vi "GPS~Logger.vi"(2 "file path (use dialog)":path, 3 "baud rate (115200)":u32=115200, 4 "stop":bool, 5 "VISA resource name":refnum<visa-resource-name>) -> (0 "Longitude":dbl format="%#_15g", 1 "Lattitude":dbl format="%#_15g")   [LabVIEW 2010]
uses:
  <vilib>/robotics/Controls/Attitude Indicator/Attitude Indicator.xctl
  <vilib>/robotics/Controls/Compass Indicator/Compass Indicator.xctl
  <vilib>/Instr/_visa.llb/VISA Set IO Buffer Mask.ctl
  <vilib>/Instr/_visa.llb/VISA Configure Serial Port (Instr).vi
panel:
  out "Bearing":dbl
  out "Speed":dbl(knob) scale=0.0..40.0
  out "LiPo":i32(slide) scale=9.0..12.6
  out "GPS Time":string
  out "Servo Roll":string
  out "Battery Voltage":dbl
  out "Distance to Waypoint":string
  out "Waypoint Number":string
  out "Flight Mode":string
  out "Compass Indicator":dbl(xcontrol)
  out "Attitude Indicator":cluster{"Roll":dbl, "Pitch":dbl}(xcontrol)
  out "Message Text":string
  in  "Tab Control":enum32{"Connectivity", "Attitude", "GPS"}(tab)
  out "error out":errorcluster {"code" format="%f"}
  out "Roll":string
  out "Pitch":string
  out "Throttle":string
  out "Airspeed":string
  out "Roll Pitch":cluster{dbl, dbl}
  out "YawNum":dbl
  out "ALT":string
  out "ALH":string
  out "BER":string
  out "CRT":string
  out "SPD":string
  out "CRS":string
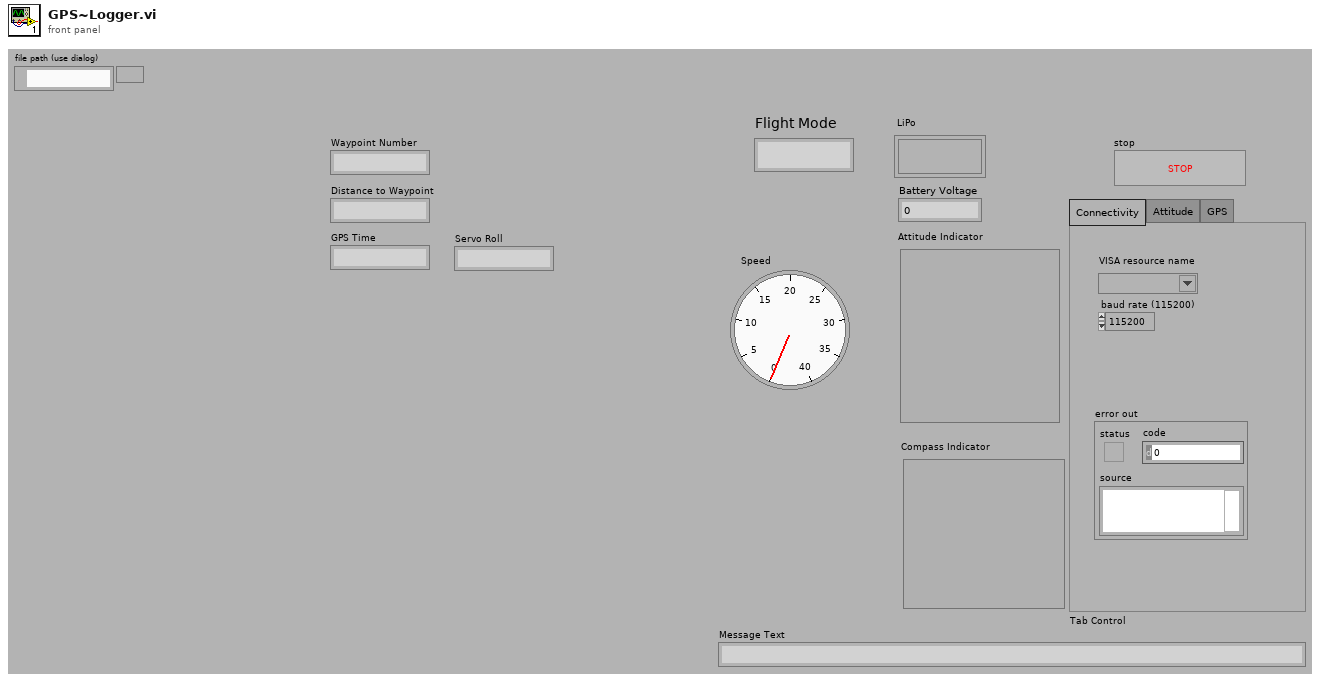
[diagram p1: front panel]
types:
  T1 = typedef "VISA Set IO Buffer Mask.ctl" = u16
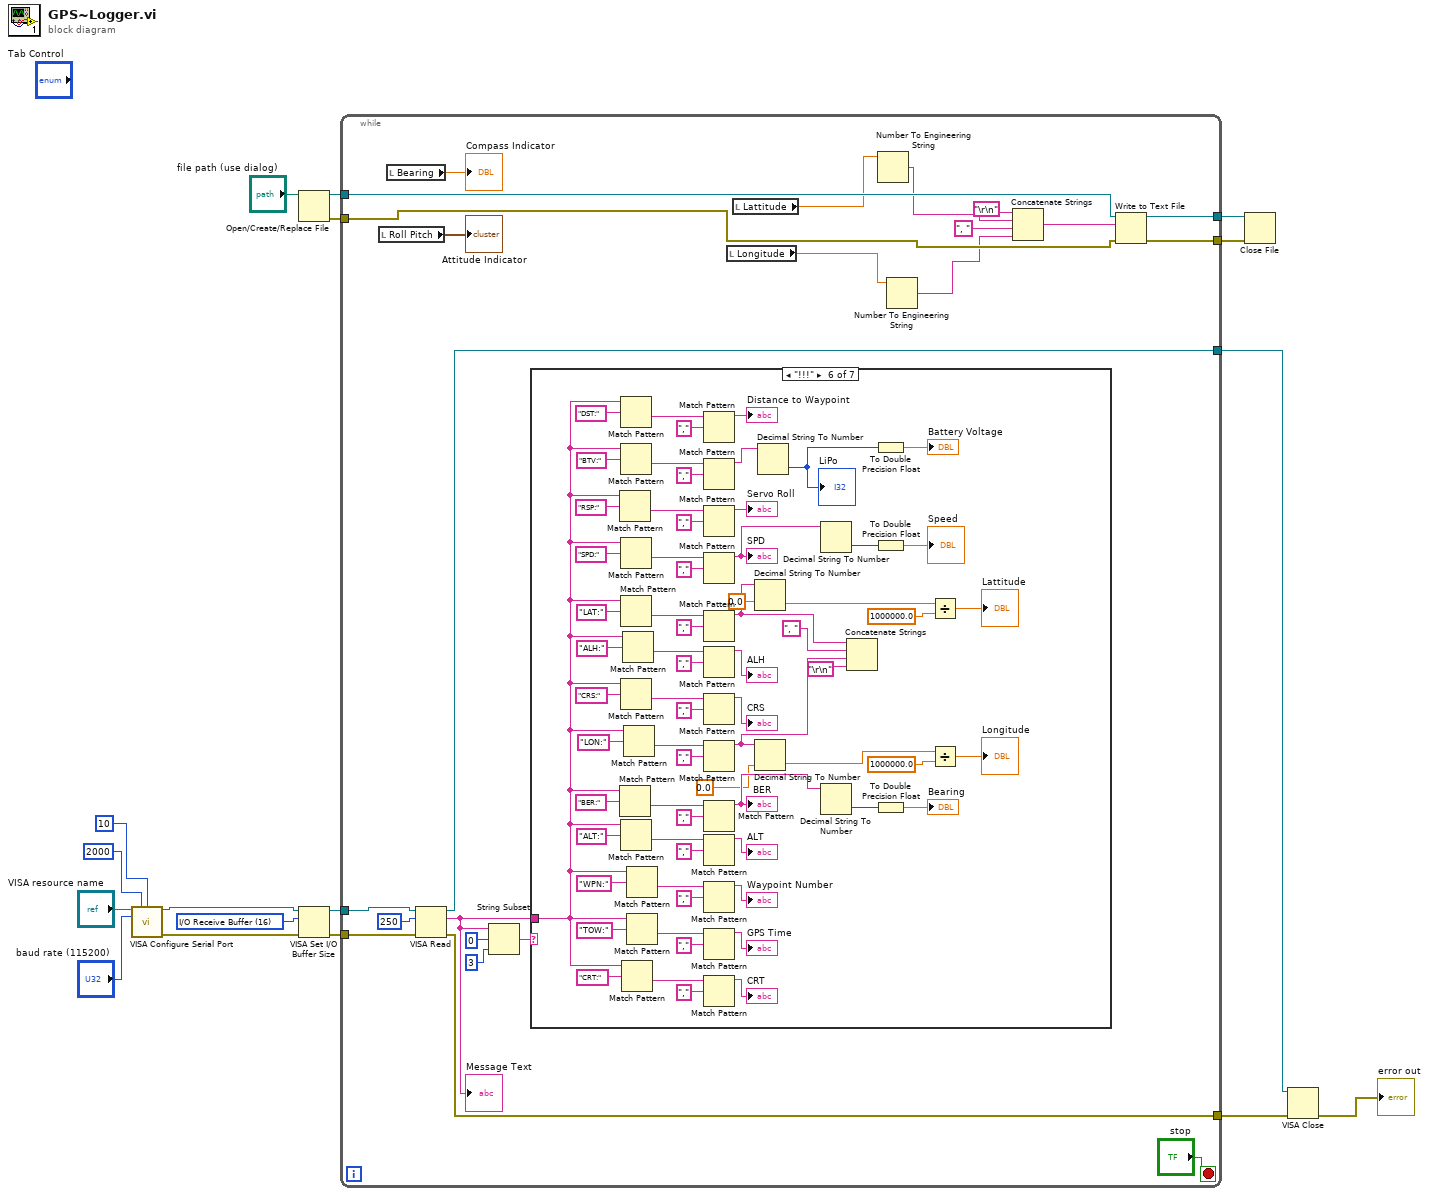
[diagram p0: block diagram]
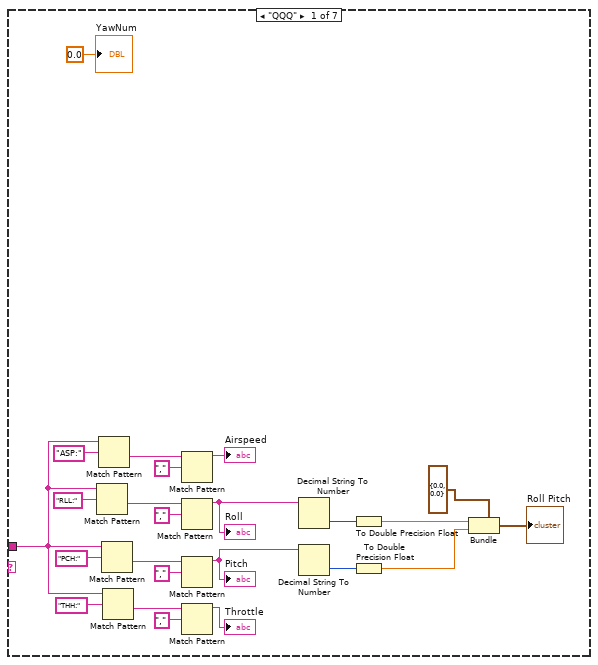
[diagram p2: hidden frame]
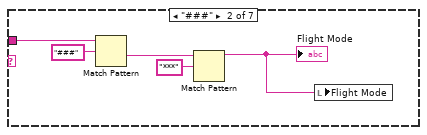
[diagram p3: hidden frame]
diagram:
  w12 = T1 16 items=["I/O Receive Buffer"=16, "I/O Transmit Buffer"=32, "I/O Receive and Transmit Buffer"=48] ("Mask")
  n1 = call-poly "VISA Configure Serial Port"("VISA resource name"="VISA resource name", "timeout (10sec)"=u32 2000, "termination char\n(0xA = '\\n' = LF)"=u8 10 ("termination char\n(0xA = '\\n' = LF)"), "baud rate (9600)"="baud rate (115200)") -> ("VISA resource name out"=w13:refnum<visa-resource-name>, "error out"=w7:errorcluster)  [unwired: 10 in]
  n2 = Open/Create/Replace File(file path (use dialog)="file path (use dialog)") -> (refnum out=w5:refnum<file>, error out=w1:errorcluster)  [unwired: 5 in, 1 out]
  n3 = VISA Set I/O Buffer Size(VISA resource name=w13, mask (16)=w12, error in (no error)=w7) -> (VISA resource name out=w11:refnum<visa-resource-name>, error out=w8:errorcluster)  [unwired: 1 in]
  n4 = while {
    tunnel: w11 -> [w40]
    tunnel: [w38] -> w10
    tunnel: [w37] -> w9
    tunnel: w8 -> [w36]
    tunnel: w5 -> [w28]
    tunnel: [w27] -> w3
    tunnel: [w24] -> w2
    tunnel: w1 -> [w23]
    stop <- "stop" stop-if-true
    n5 = local read "Roll Pitch"() -> (→"Attitude Indicator":cluster{dbl, dbl})
    n6 = local read "Bearing"() -> (→"Compass Indicator":dbl)
    n7 = VISA Read(VISA resource name=w40, byte count=u32 250, error in (no error)=w36) -> (VISA resource name out=w38:refnum<visa-resource-name>, read buffer=w30:string, error out=w37:errorcluster)  [unwired: 1 out]
    "Message Text" <- w30
    n8 = String Subset(string=w30, offset (0)=0, length (rest)=3 ("length (rest)")) -> (substring=w29:string)
    n9 = case shown="\"!!!\"" w29 {
      tunnel: w30 -> [w42 w69 _ _ _ w90 _]
      frame "QQQ" {
        n10 = Match Pattern(string=w42, regular expression="RLL:") -> (after substring=w63:string)  [unwired: 4 out]
        n11 = Match Pattern(string=w42, regular expression="ASP:") -> (after substring=w54:string)  [unwired: 4 out]
        n12 = Match Pattern(string=w42, regular expression="PCH:") -> (after substring=w60:string)  [unwired: 4 out]
        n13 = Match Pattern(string=w42, regular expression="THH:") -> (after substring=w57:string)  [unwired: 4 out]
        n14 = Match Pattern(string=w54, regular expression=",") -> (before substring=→"Airspeed":string)  [unwired: 4 out]
        n15 = Match Pattern(string=w63, regular expression=",") -> (before substring=w45:string)  [unwired: 4 out]
        "Roll" <- w45
        n16 = Match Pattern(string=w60, regular expression=",") -> (before substring=w44:string)  [unwired: 4 out]
        "Pitch" <- w44
        n17 = Match Pattern(string=w57, regular expression=",") -> (before substring=→"Throttle":string)  [unwired: 4 out]
        n18 = Decimal String To Number(string=w45) -> (number=w51:i32)  [unwired: 2 in, 1 out]
        n19 = Decimal String To Number(string=w44) -> (number=w50:i32)  [unwired: 2 in, 1 out]
        n20 = To Double Precision Float(number=w51) -> (double precision float=w48:dbl)
        n21 = To Double Precision Float(number=w50) -> (double precision float=w49:dbl)
        n22 = Bundle(cluster=cluster{dbl, dbl} {0.0, 0.0} ("Cluster"), w48, w49) -> (→"Roll Pitch":cluster{dbl, dbl})
        "YawNum" <- 0.0 ("YawNum")
      }
      frame "###" {
        n23 = Match Pattern(string=w69, regular expression="###") -> (after substring=w67:string)  [unwired: 1 in, 3 out]
        n24 = Match Pattern(string=w67, regular expression="***") -> (before substring=w65:string)  [unwired: 1 in, 3 out]
        "Flight Mode" <- w65
        n25 = local write "Flight Mode"(w65) -> ()
      }
      frame "%%%" {
      }
      frame "XXX" {
      }
      frame "PPP" {
      }
      frame "!!!" {
        n26 = Match Pattern(string=w90, regular expression="RSP:") -> (after substring=w97:string)  [unwired: 4 out]
        n27 = Match Pattern(string=w90, regular expression="BER:") -> (after substring=w117:string)  [unwired: 4 out]
        n28 = Match Pattern(string=w90, regular expression="DST:") -> (after substring=w104:string)  [unwired: 4 out]
        n29 = Match Pattern(string=w90, regular expression="BTV:") -> (after substring=w100:string)  [unwired: 4 out]
        n30 = Match Pattern(string=w90, regular expression="SPD:") -> (after substring=w127:string)  [unwired: 4 out]
        n31 = Match Pattern(string=w90, regular expression="LAT:") -> (after substring=w137:string)  [unwired: 4 out]
        n32 = Match Pattern(string=w90, regular expression="CRS:") -> (after substring=w120:string)  [unwired: 4 out]
        n33 = Match Pattern(string=w90, regular expression="ALT:") -> (after substring=w131:string)  [unwired: 4 out]
        n34 = Match Pattern(string=w90, regular expression="CRT:") -> (after substring=w124:string)  [unwired: 4 out]
        n35 = Match Pattern(string=w90, regular expression="ALH:") -> (after substring=w114:string)  [unwired: 4 out]
        n36 = Match Pattern(string=w90, regular expression="LON:") -> (after substring=w134:string)  [unwired: 4 out]
        n37 = Match Pattern(string=w90, regular expression="WPN:") -> (after substring=w108:string)  [unwired: 4 out]
        n38 = Match Pattern(string=w90, regular expression="TOW:") -> (after substring=w93:string)  [unwired: 4 out]
        n39 = Match Pattern(string=w104, regular expression=",") -> (before substring=→"Distance to Waypoint":string)  [unwired: 4 out]
        n40 = Match Pattern(string=w100, regular expression=",") -> (before substring=w89:string)  [unwired: 4 out]
        n41 = Match Pattern(string=w97, regular expression=",") -> (before substring=→"Servo Roll":string)  [unwired: 4 out]
        n42 = Match Pattern(string=w127, regular expression=",") -> (before substring=w84:string)  [unwired: 4 out]
        "SPD" <- w84
        n43 = Match Pattern(string=w137, regular expression=",") -> (before substring=w79:string)  [unwired: 4 out]
        n44 = Match Pattern(string=w114, regular expression=",") -> (before substring=→"ALH":string)  [unwired: 4 out]
        n45 = Match Pattern(string=w120, regular expression=",") -> (before substring=→"CRS":string)  [unwired: 4 out]
        n46 = Match Pattern(string=w134, regular expression=",") -> (before substring=w75:string)  [unwired: 4 out]
        n47 = Match Pattern(string=w117, regular expression=",") -> (before substring=w80:string)  [unwired: 4 out]
        "BER" <- w80
        n48 = Match Pattern(string=w131, regular expression=",") -> (before substring=→"ALT":string)  [unwired: 4 out]
        n49 = Match Pattern(string=w108, regular expression=",") -> (before substring=→"Waypoint Number":string)  [unwired: 4 out]
        n50 = Match Pattern(string=w93, regular expression=",") -> (before substring=→"GPS Time":string)  [unwired: 4 out]
        n51 = Match Pattern(string=w124, regular expression=",") -> (before substring=→"CRT":string)  [unwired: 4 out]
        n52 = Decimal String To Number(string=w79, default (0L)=0.0 ("default (0 I32)")) -> (number=w72:dbl)  [unwired: 1 in, 1 out]
        n53 = Decimal String To Number(string=w75, default (0L)=0.0 ("default (0 I32)")) -> (number=w70:dbl)  [unwired: 1 in, 1 out]
        n54 = Decimal String To Number(string=w89) -> (number=w87:i32)  [unwired: 2 in, 1 out]
        "LiPo" <- w87
        n55 = Decimal String To Number(string=w84) -> (number=w85:i32)  [unwired: 2 in, 1 out]
        n56 = Decimal String To Number(string=w80) -> (number=w83:i32)  [unwired: 2 in, 1 out]
        n57 = Concatenate Strings(w79, ", " ("string"), w75, "\r\n") -> ()  [unwired: 1 out]
        n58 = To Double Precision Float(number=w87) -> (double precision float=→"Battery Voltage":dbl)
        n59 = To Double Precision Float(number=w85) -> (double precision float=→"Speed":dbl)
        n60 = To Double Precision Float(number=w83) -> (double precision float=→"Bearing":dbl)
        n61 = Divide(x=w72, y=1000000.0) -> (x/y=→"Lattitude":dbl)
        n62 = Divide(x=w70, y=1000000.0) -> (x/y=→"Longitude":dbl)
      }
      frame Default {
      }
    }
    n63 = local read "Longitude"() -> (w21:dbl)
    n64 = local read "Lattitude"() -> (w18:dbl)
    n65 = Number To Engineering String(4:w18) -> (0:w19:string)  [unwired: 3 in]
    n66 = Number To Engineering String(4:w21) -> (0:w20:string)  [unwired: 3 in]
    n67 = Concatenate Strings("\r\n", w19, ", " ("string"), w20) -> (w26:string)
    n68 = Write to Text File(file (use dialog)=w28, text=w26, error in=w23) -> (refnum out=w27:refnum<file>, error out=w24:errorcluster)  [unwired: 1 in, 1 out]
  }
  n69 = Close File(refnum=w3, error in=w2) -> ()  [unwired: 2 out]
  n70 = VISA Close(VISA resource name=w10, error in (no error)=w9) -> (error out=→"error out":errorcluster)
